vi "Query - String - Scalar.vi"(8 "error in":errorcluster, 10 "Query":string, 11 "Module ID":i32=-1) -> (0 "error out":errorcluster, 1 "Meta Data":variant, 2 "Return Data":string, 4 "Field Names":string[](array[string]))   [LabVIEW 2014, in "DB_CONNECTOR.lvlib"]
uses:
  DB_CONNECTOR.lvlib
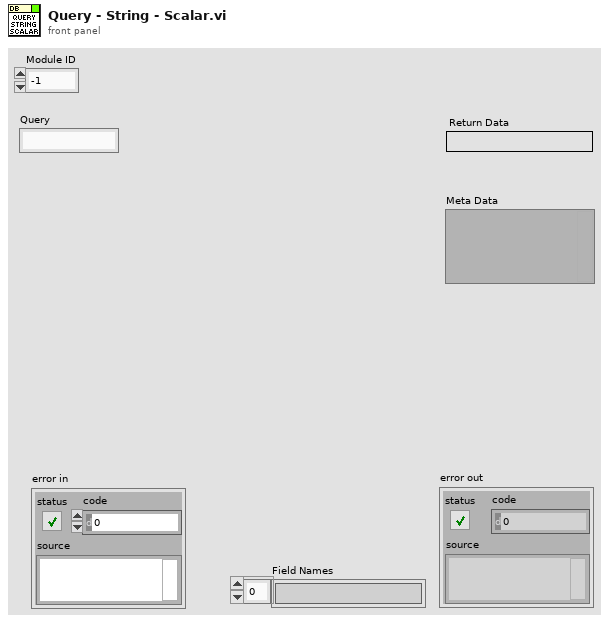
[diagram p1: front panel]
types:
  T1 = typedef "DB_CONNECTOR.lvlib/Query (Reply Payload)--cluster.ctl" = cluster{"Return Data":string[][], "Meta Data":variant, "Field Names":string[], "Query_error":errorcluster}
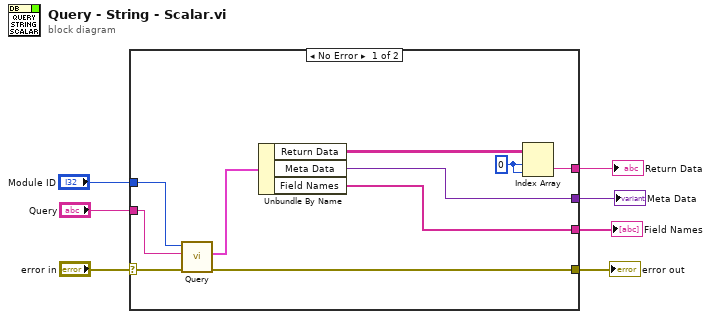
[diagram p0: block diagram]
diagram:
  n1 = case shown="No Error" "error in" {
    selector: "error in" -> [w17 w18]
    tunnel: [w10 w18] -> w6
    tunnel: "Query" -> [w9 _]
    tunnel: "Module ID" -> [w15 _]
    tunnel: [w13 _] -> w2
    tunnel: [w11 _] -> w3
    tunnel: [w8 _] -> w1
    frame No Error {
      w12 = 0 ("index (row)")
      n2 = call "Query.vi"("error in (no error)"=w17, "Query"=w9, "Module ID"=w15) -> ("error out"=w10:errorcluster, "Reply Payload"=w16:T1)  [unwired: 7 in]
      n3 = Unbundle By Name(w16) -> ("Return Data"=w14:string[][], "Meta Data"=w13:variant, "Field Names"=w8:string[])
      n4 = Index Array(array=w14, index (row)=w12, index (col)=w12) -> (element=w11:string)
    }
    frame Error {
    }
  }
  "error out" <- w6
  "Return Data" <- w3
  "Meta Data" <- w2
  "Field Names" <- w1
